vi "Configure Measurement Filter.vi"(5 "Window":dbl max=10.0, 6 "Number of Filter Readings (10)":u32 min=1 max=100, 7 "Filter Type":u16(ring) items=["Repeating", "Moving"], 8 "error in (no error)":errorcluster, 9 "Enable Filter  (T: Enable)":bool, 10 "Function":u16(ring) items=["Voltage: DC", "Voltage: AC", "Current: DC", "Current: AC", "2W Resistance", "4W Resistance", "Diode", "Capacitance", "Temperature", "Continuity", "Frequency", "Period", "Ratio", "Digitize Voltage", "Digitize Current"], 11 "VISA resource name":refnum<visa-resource-name>) -> (0 "error out":errorcluster, 3 "VISA resource name out":refnum<visa-resource-name>)   [LabVIEW 2009, in "Keithley DMM7510.lvlib"]
doc: "Configures the measurement filter, including the number of readings averaged the type of filter applied."
uses:
  Keithley DMM7510.lvlib
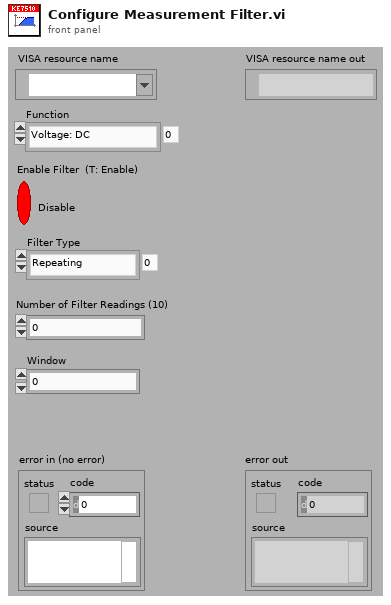
[diagram p1: front panel]
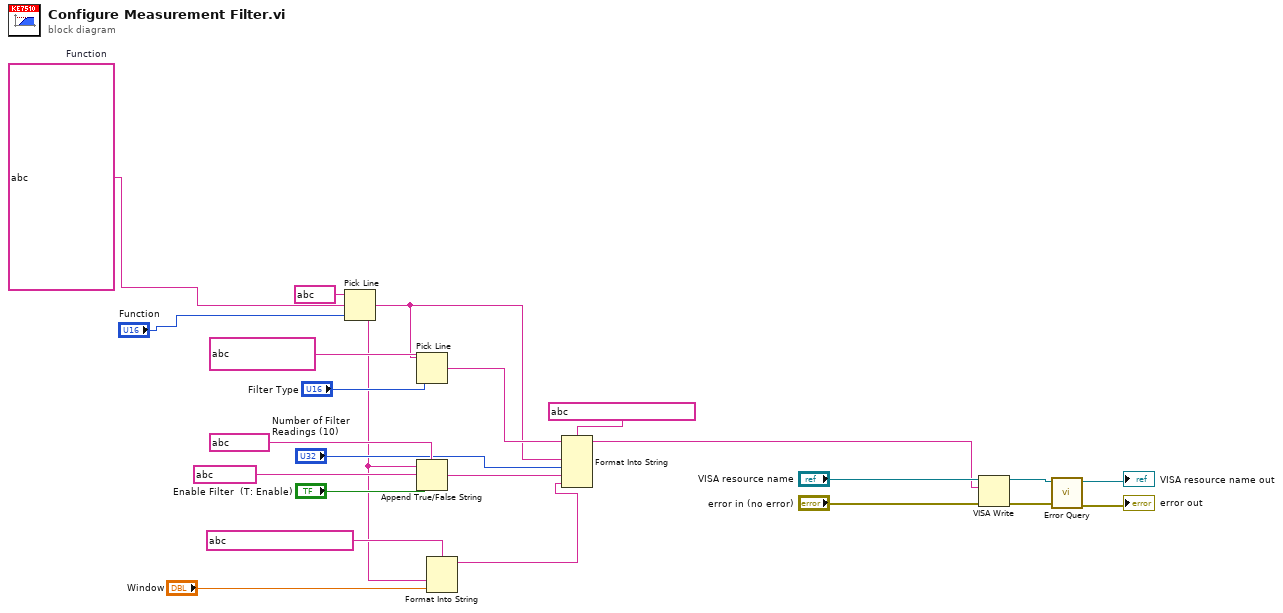
[diagram p0: block diagram]
diagram:
  w2 = string ?  # Function
  n1 = Pick Line(string ("")=string ?, multi-line string=w2, line index="Function") -> (output string=w10:string)
  n2 = Pick Line(string ("")=w10, multi-line string=string ?, line index="Filter Type") -> (output string=w12:string)
  n3 = Append True/False String(1:"Enable Filter  (T: Enable)", 2:string ?, 3:string ?, 4:w10) -> (0:w14:string)
  n4 = Format Into String(format string=string ?, w10, "Window") -> (resulting string=w8:string)  [unwired: 2 in, 1 out]
  n5 = Format Into String(format string=string ?, initial string=w12, w10, "Number of Filter Readings (10)", w14, w8) -> (resulting string=w18:string)  [unwired: 1 in, 1 out]
  n6 = VISA Write(VISA resource name="VISA resource name", write buffer=w18, error in (no error)="error in (no error)") -> (VISA resource name out=w7:refnum<visa-resource-name>, error out=w6:errorcluster)  [unwired: 1 out]
  n7 = call "Error Query.vi"("error in (no error)"=w6, "VISA resource name"=w7) -> ("error out"=→"error out":errorcluster, "VISA resource name out"=→"VISA resource name out":refnum<visa-resource-name>)  [unwired: 8 out]
